vi "ensender y apagar un led.vi"() -> ()   [LabVIEW 2016]
uses:
  <vilib>/LabVIEW Interface for Arduino/Type Defs/Board Type.ctl
  <vilib>/LabVIEW Interface for Arduino/Type Defs/Connection Type.ctl
  <vilib>/LabVIEW Interface for Arduino/LabVIEW Interface for Arduino.lvlib
panel:
  out "Estado":u32
  in  "stop":bool
  out "Led":bool
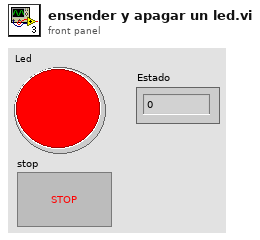
[diagram p1: front panel]
types:
  T1 = typedef "LabVIEW Interface for Arduino.lvlib/Connection Type.ctl" = enum8{"USB / Serial", "XBEE", "BlueSmirf (Bluetooth)"}
  T2 = typedef "LabVIEW Interface for Arduino.lvlib/Board Type.ctl" = enum16{"Uno", "Dimuelanove w/Atmega 328", "Mega 2560"}
  T3 = typedef "LabVIEW Interface for Arduino.lvlib/Arduino Resource.ctl" = cluster{"VISA resource":refnum<visa-resource-name>, "Board Type":T2, "Connection Type":enum8{"USB / Serial"}, "Bytes Per Packet (15)":u8}
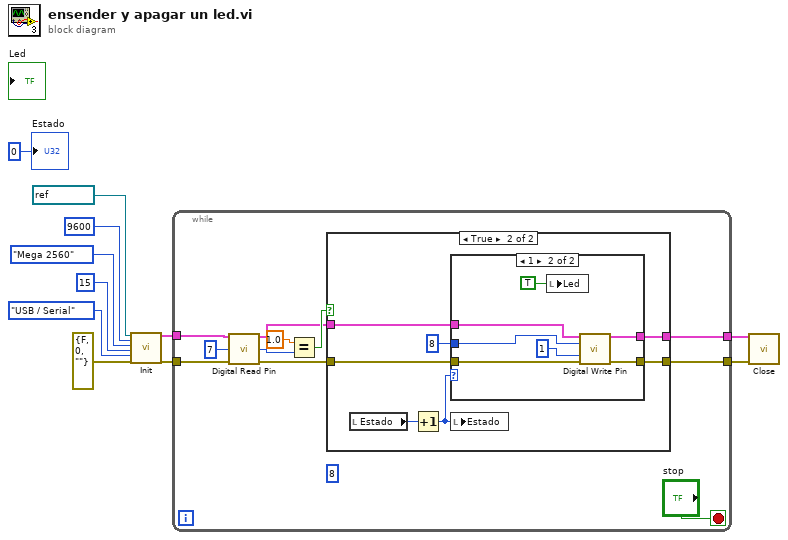
[diagram p0: block diagram]
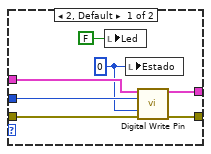
[diagram p3: hidden frame]
diagram:
  n1 = call <vilib>:"Init.vi"("VISA resource"=refnum<visa-resource-name> "COM6", "Baud Rate (115200)"=u32 9600, "Board Type (Uno)"=Board_Type."Mega 2560", "Bytes Per Packet (15)"=u32 15, "Connection Type (USB/Serial)"=Connection_Type."USB / Serial", "error in"=errorcluster {"status"=FALSE, "code"=0, "source"=""}) -> ("Arduino Resource"=w11:T3, "error out"=w10:errorcluster)  [unwired: 12 in]
  n2 = while {
    tunnel: w11 -> [w22]
    tunnel: w10 -> [w21]
    tunnel: [w13] -> w3
    tunnel: [w12] -> w2
    stop <- "stop" stop-if-true
    (unwired) u8 8 ("Digital I/O Pin (0)")
    n3 = call <vilib>:"Digital Read Pin.vi"("Arduino Resource"=w22, "Digital I/O Pin (0)"=u8 7, "error in"=w21) -> ("Arduino Resource"=w15:T3, "Value"=w17:u8, "error out"=w14:errorcluster)  [unwired: 10 in]
    n4 = Equal?(x=1.0, y=w17) -> (x = y?=w16:bool)
    n5 = case shown="True" w16 {
      tunnel: w15 -> [w23 w29]
      tunnel: w14 -> [w24 w28]
      tunnel: [w23 w26] -> w13
      tunnel: [w24 w25] -> w12
      frame False {
      }
      frame True {
        n6 = local read "Estado"() -> (w31:u32)
        n7 = Increment(x=w31) -> (x+1=w30:u32)
        n8 = case shown="1" w30 {
          tunnel: w29 -> [w37 w45]
          tunnel: w28 -> [w36 w44]
          tunnel: u8 8 ("Digital I/O Pin (0)") -> [w33 w43]
          tunnel: [w35 w41] -> w26
          tunnel: [w34 w40] -> w25
          frame 2, Default {
            w32 = u8 0 ("Value (0)")
            n9 = local write "Led"(FALSE ("Led")) -> ()
            n10 = local write "Estado"(w32) -> ()
            n11 = call <vilib>:"Digital Write Pin.vi"("Arduino Resource"=w37, "Digital I/O Pin (0)"=w33, "Value (0)"=w32, "error in"=w36) -> ("Arduino Resource"=w35:T3, "error out"=w34:errorcluster)  [unwired: 10 in]
          }
          frame 1 {
            n12 = local write "Led"(TRUE ("Led")) -> ()
            n13 = call <vilib>:"Digital Write Pin.vi"("Arduino Resource"=w45, "Digital I/O Pin (0)"=w43, "Value (0)"=u8 1, "error in"=w44) -> ("Arduino Resource"=w41:T3, "error out"=w40:errorcluster)  [unwired: 10 in]
          }
        }
        n14 = local write "Estado"(w30) -> ()
      }
    }
  }
  n15 = call <vilib>:"Close.vi"("Arduino Resource"=w3, "error in"=w2) -> ()  [unwired: 13 in, 1 out]
  "Estado" <- u32 0 ("Estado")
